vi "Create or Substitute NI_Layer layer.vi"(1 "All Layers in":refnum<class "Layer.lvclass">[](array[class]), 2 "new picture":picture) -> (0 "All Layers out":refnum<class "Layer.lvclass">[](array[class]))   [LabVIEW 2020]
uses:
  vi.lib/LabVIEW Icon API/lv_icon/Classes/Layer/Layer.lvclass
  vi.lib/LabVIEW Icon API/lv_icon/Controls/Layer.ctl
  vi.lib/LabVIEW Icon API/lv_icon/lv_icon.lvlib
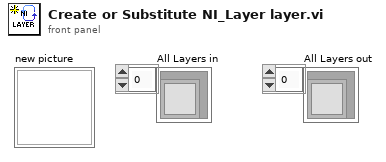
[diagram p1: front panel]
types:
  T1 = typedef "Layer.ctl" = cluster{"LayerIcon":picture, "LayerName":string, "Opacity":u8, "Visibility?":bool}
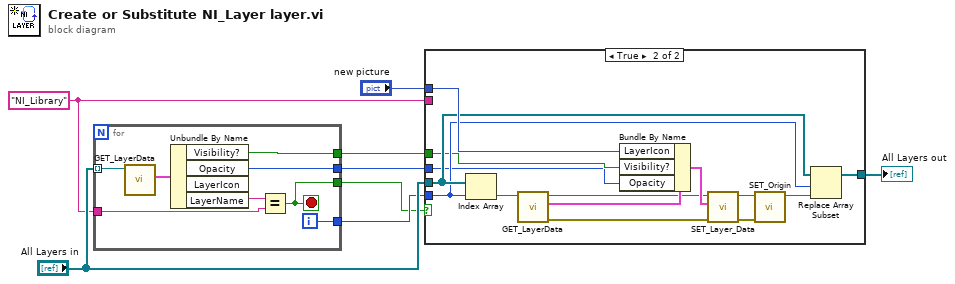
[diagram p0: block diagram]
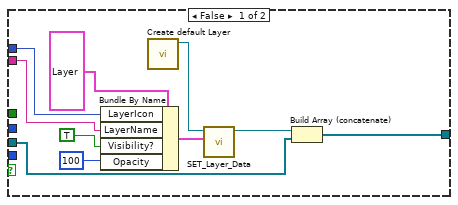
[diagram p2: hidden frame]
diagram:
  w4 = "NI_Library" ("LayerName")
  n1 = for {
    tunnel: "All Layers in" -> [w16] mode=indexing
    tunnel: [w13] -> w3
    tunnel: [w12] -> w1
    tunnel: w4 -> [w11]
    tunnel: [w10] -> w6
    tunnel: [w9] -> w5
    i -> [w13]
    stop <- w12 stop-if-true
    n2 = call-dynamic "GET_LayerData.vi"("Layer.lvclass in"=w16) -> ("Data"=w15:T1)  [unwired: 1 in, 9 out]
    n3 = Unbundle By Name(w15) -> ("Visibility?"=w9:bool, "Opacity"=w10:u8, "LayerName"=w14:string)  [unwired: 1 out]
    n4 = Equal?(x=w14, y=w11) -> (x = y?=w12:bool)
  }
  n5 = case shown="True" w1 {
    tunnel: "All Layers in" -> [w26 w32]
    tunnel: "new picture" -> [w24 w36]
    tunnel: w3 -> [_ w30]
    tunnel: [w22 w29] -> w7
    tunnel: w4 -> [w19 _]
    tunnel: w5 -> [_ w28]
    tunnel: w6 -> [_ w27]
    frame False {
      n6 = Bundle By Name(cluster=T1 {"LayerIcon"=bytes[0], "LayerName"="", "Opacity"=0, "Visibility?"=FALSE} ("Data"), "LayerIcon"=w24, "LayerName"=w19, "Visibility?"=TRUE, "Opacity"=u8 100) -> (w23:T1)
      n7 = call "Create default Layer.vi"() -> ("Layer.lvclass out"=w21:refnum<class "Layer.lvclass">)  [unwired: 1 in, 10 out]
      n8 = call-dynamic "SET_Layer_Data.vi"("Data"=w23, "Layer.lvclass in"=w21) -> ("Layer.lvclass out"=w25:refnum<class "Layer.lvclass">)  [unwired: 2 in, 7 out]
      n9 = Build Array (concatenate)(w25, w26) -> (w22:refnum<class "Layer.lvclass">[])
    }
    frame True {
      n10 = Index Array(array=w32, index=w30) -> (element=w40:refnum<class "Layer.lvclass">)
      n11 = call-dynamic "GET_LayerData.vi"("Layer.lvclass in"=w40) -> ("error out"=w33:errorcluster, "Data"=w37:T1, "Layer.lvclass out"=w34:refnum<class "Layer.lvclass">)  [unwired: 1 in, 7 out]
      n12 = Bundle By Name(cluster=w37, "LayerIcon"=w36, "Visibility?"=w28, "Opacity"=w27) -> (w35:T1)
      n13 = call-dynamic "SET_Layer_Data.vi"("error in (no error)"=w33, "Data"=w35, "Layer.lvclass in"=w34) -> ("error out"=w38:errorcluster, "Layer.lvclass out"=w39:refnum<class "Layer.lvclass">)  [unwired: 1 in, 6 out]
      n14 = call-dynamic "SET_Origin.vi"("error in"=w38, "Layer.lvclass in"=w39) -> ("Layer.lvclass out"=w31:refnum<class "Layer.lvclass">)  [unwired: 1 in, 8 out]
      n15 = Replace Array Subset(array=w32, new element=w31, index=w30) -> (w29:refnum<class "Layer.lvclass">[])
    }
  }
  "All Layers out" <- w7
